vi "Teleop Drivetrain Control.vi"(9 "D-Pad":T1, 10 "Button Cluster":T2, 11 "Axes":T3) -> ()   [LabVIEW 2016]
uses:
  Robot Global Data.vi
  Common Code/Drive Mode.ctl
  Common Code/Gamepads/Axes Cluster.ctl
  Common Code/Gamepads/Button Cluster.ctl
  Common Code/Gamepads/D-Pad.ctl
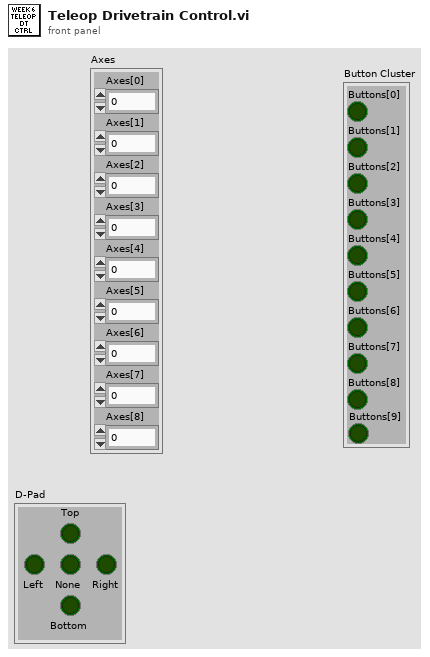
[diagram p1: front panel]
types:
  T1 = typedef "D-Pad.ctl" = cluster{"Top":bool, "Bottom":bool, "None":bool, "Right":bool, "Left":bool}
  T2 = typedef "Button Cluster.ctl" = cluster{"Buttons[0]":bool, "Buttons[1]":bool, "Buttons[2]":bool, "Buttons[3]":bool, "Buttons[4]":bool, "Buttons[5]":bool, "Buttons[6]":bool, "Buttons[7]":bool, "Buttons[8]":bool, "Buttons[9]":bool}
  T3 = typedef "Axes Cluster.ctl" = cluster{"Axes[0]":dbl, "Axes[1]":dbl, "Axes[2]":dbl, "Axes[3]":dbl, "Axes[4]":dbl, "Axes[5]":dbl, "Axes[6]":dbl, "Axes[7]":dbl, "Axes[8]":dbl}
  T4 = typedef "Drive Mode.ctl" = enum16{"Gyro Steer", "Manual"}
  T5 = typedef "Drivetrain Command Cluster.ctl" = cluster{"Y Max Output":dbl, "Y Min Output":dbl, "X Max Output":dbl, "X Min Output":dbl, "Heading Target":dbl, "Turn Power":dbl, "Y Power":dbl, "Drive Mode":T4}
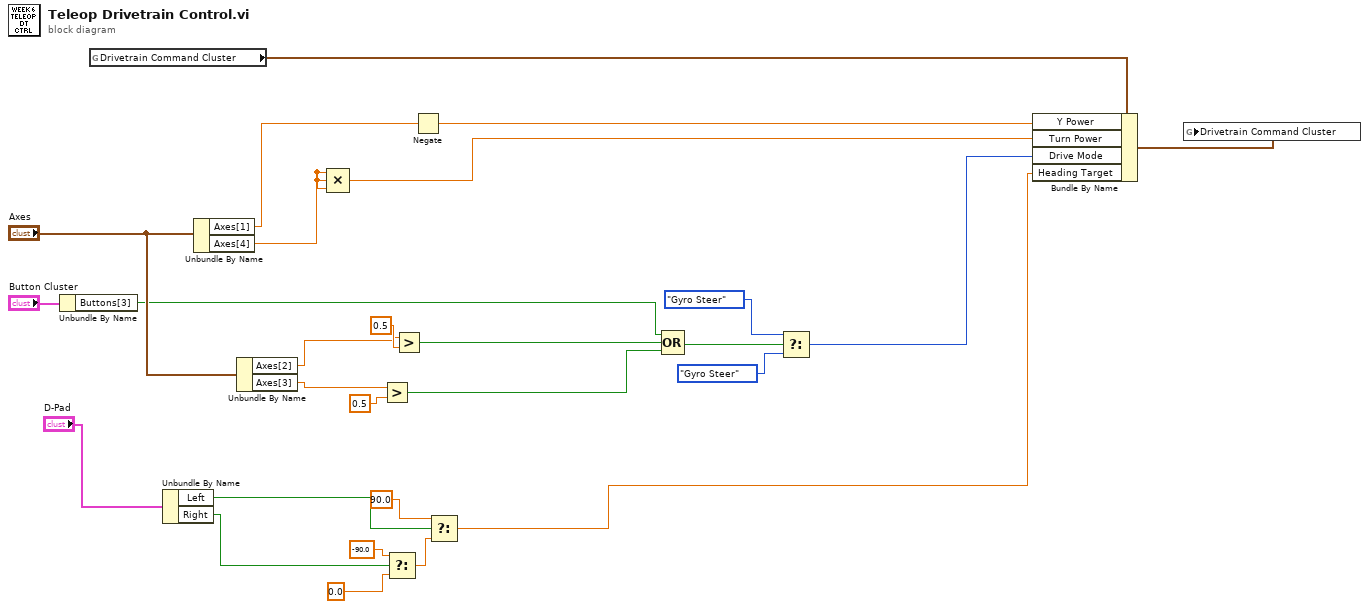
[diagram p0: block diagram]
diagram:
  n1 = Unbundle By Name("Button Cluster") -> ("Buttons[3]"=w15:bool)
  n2 = global read "Robot Global Data.vi" "Drivetrain Command Cluster"() -> (w26:T5)
  n3 = Unbundle By Name("D-Pad") -> ("Left"=w5:bool, "Right"=w4:bool)
  n4 = Unbundle By Name("Axes") -> ("Axes[1]"=w23:dbl, "Axes[4]"=w27:dbl)
  n5 = Unbundle By Name("Axes") -> ("Axes[2]"=w18:dbl, "Axes[3]"=w17:dbl)
  n6 = Compound Arithmetic op=MULTIPLY(w27, w27, w27) -> (w22:dbl)
  n7 = Greater?(x=w17, y=0.5) -> (0:w13:bool)
  n8 = Select(t=-90.0, s=w4, f=0.0) -> (s? t:f=w3:dbl)
  n9 = Greater?(x=w18, y=0.5) -> (0:w14:bool)
  n10 = Negate(x=w23) -> (-x=w24:dbl)
  n11 = Select(t=90.0, s=w5, f=w3) -> (s? t:f=w1:dbl)
  n12 = Compound Arithmetic op=OR(w15, w14, w13) -> (w12:bool)
  n13 = Select(t=Drive_Mode."Gyro Steer" ("Drive Mode"), s=w12, f=Drive_Mode."Gyro Steer" ("Drive Mode")) -> (s? t:f=w9:T4)
  n14 = Bundle By Name(cluster=w26, "Y Power"=w24, "Turn Power"=w22, "Drive Mode"=w9, "Heading Target"=w1) -> (w25:T5)
  n15 = global write "Robot Global Data.vi" "Drivetrain Command Cluster"(w25) -> ()
